vi "CALL_WT230.vi"(11 "simulazione":bool) -> ()   [LabVIEW 2019]
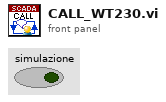
[diagram p1: front panel]
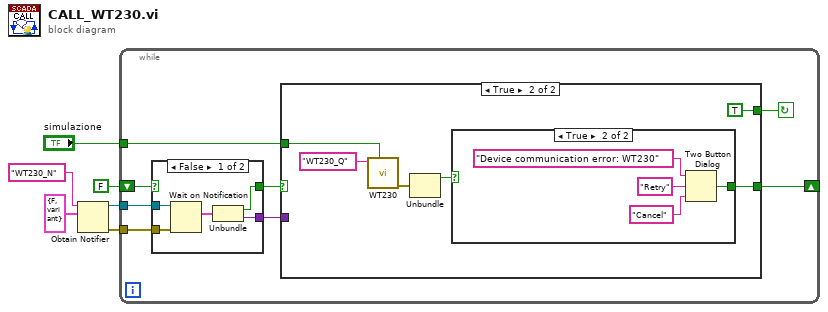
[diagram p0: block diagram]
diagram:
  n1 = Obtain Notifier(name (unnamed)="WT230_N" ("Notifier Name"), notification data type=cluster{"boolean":bool, "variant":variant} {"boolean"=FALSE, "variant"=variant} ("notification")) -> (notifier out=w4:refnum<notifier>, error out=w5:errorcluster)  [unwired: 2 in, 1 out]
  n2 = while {
    tunnel: "simulazione" -> [w13]
    tunnel: w5 -> [w11]
    tunnel: w4 -> [w12]
    shift-right: [w7] -> _
    shift-left: FALSE -> [w8]
    stop <- w14 continue-if-true
    n3 = case shown="False" w8 {
      selector: w8 -> [_ w20]
      tunnel: w12 -> [w19 _]
      tunnel: w11 -> [w18 _]
      tunnel: [w16 w20] -> w10
      tunnel: [w15 _] -> w9
      frame False {
        n4 = Wait on Notification(notifier=w19, error in (no error)=w18) -> (notification=w17:cluster{"boolean":bool, "variant":variant})  [unwired: 2 in, 3 out]
        n5 = Unbundle(w17) -> ("boolean"=w16:bool, "variant"=w15:variant)
      }
      frame True {
      }
    }
    n6 = case shown="True" w10 {
      selector: w10 -> [w21 _]
      tunnel: [w21 TRUE] -> w14
      tunnel: w9 -> [_ _]
      tunnel: w13 -> [_ w26]
      tunnel: [_ w23] -> w7
      frame False {
      }
      frame True {
        n7 = call "WT230.vi"("simulazione"=w26, "Queue Name"="WT230_Q") -> ("error out"=w27:errorcluster)  [unwired: 8 in, 1 out]
        n8 = Unbundle(w27) -> ("status"=w24:bool)  [unwired: 2 out]
        n9 = case shown="True" w24 {
          tunnel: [_ w28] -> w23
          frame False {
          }
          frame True {
            n10 = Two Button Dialog(message="Device communication error: WT230", 1:"Cancel" ("Right Button Text (\"Cancel\")"), 2:"Retry" ("Left Button Text (\"Yes\")")) -> (T button?=w28:bool)
          }
        }
      }
    }
  }
